vi "CloseMUXChannel.vi"(8 "error in (no error)":errorcluster, 10 "gRPCid":T2, 11 "ctet_mux in":T1) -> (0 "error out":errorcluster, 3 "ctet_mux out":T1)   [LabVIEW 2019, in "ctet_mux_User Library.lvlib"]
uses:
  ctet_mux_User Library.lvlib
  Servers/ctet_mux/gRPC lvSupport/Server API/typeDefs/grpcId.ctl
  Types/ctet_mux.ctl
  Servers/ctet_mux/ctet_mux Class/RPC Messages/measurementservice_MUXCloseChannelResponse/measurementservice_MUXCloseChannelResponse_Data.ctl
  Servers/ctet_mux/ctet_mux Class/RPC Messages/measurementservice_ErrorOut/measurementservice_ErrorOut_Data.ctl
  <instrlib>/niSwitch/niSwitch.llb/niSwitch Connect Channels (Single).vi
  Servers/ctet_mux/ctet_mux Class/ctet_mux.lvclass
  Servers/ctet_mux/gRPC lvSupport/gprc-lvsupport.lvlib
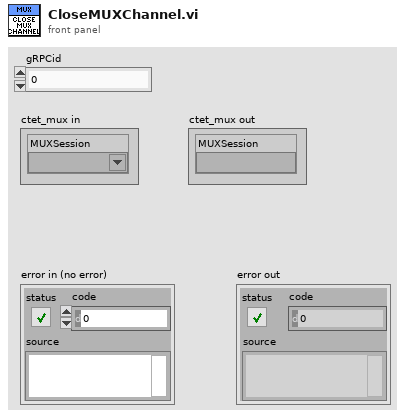
[diagram p1: front panel]
types:
  T1 = typedef "ctet_mux_User Library.lvlib/ctet_mux.ctl" = cluster{"MUXSession":refnum<k15>}
  T2 = typedef "ctet_mux.lvlib/gprc-lvsupport.lvlib/grpcId.ctl" = u64
  T3 = typedef "ctet_mux.lvlib/ctet_mux.lvclass/measurementservice_ErrorOut_Data.ctl" = cluster{"errCode":i64, "errMessage":string}
  T4 = typedef "ctet_mux.lvlib/ctet_mux.lvclass/measurementservice_MUXCloseChannelResponse_Data.ctl" = cluster{"error":T3}
  T5 = typedef "ctet_mux.lvlib/ctet_mux.lvclass/measurementservice_MUXCloseChannelRequest_Data.ctl" = cluster{"Channel1":string, "Channel2":string}
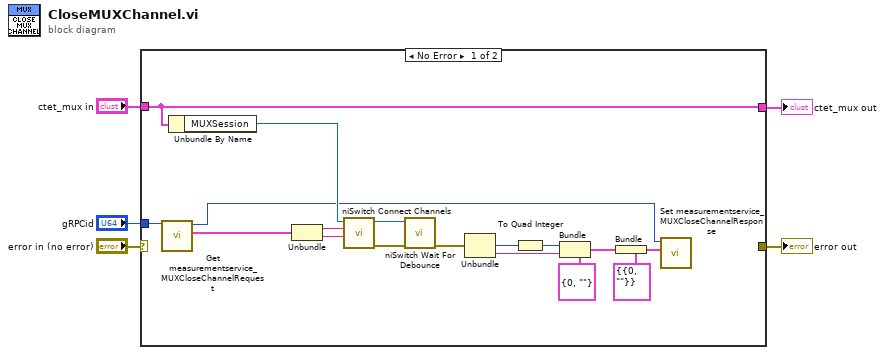
[diagram p0: block diagram]
diagram:
  n1 = case shown="No Error" "error in (no error)" {
    selector: "error in (no error)" -> [_ w24]
    tunnel: [_ w24] -> w5
    tunnel: "gRPCid" -> [w18 _]
    tunnel: "ctet_mux in" -> [w19 w23]
    tunnel: [w19 w23] -> w1
    frame No Error {
      n2 = call "Get measurementservice_MUXCloseChannelRequest.vi"("gRPCid"=w18) -> ("Message Data"=w17:T5, "gRPCid out"=w6:T2)  [unwired: 8 in, 1 out]
      n3 = Unbundle By Name(w19) -> ("MUXSession"=w9:refnum<k15>)
      n4 = Unbundle(w17) -> ("Channel1"=w8:string, "Channel2"=w7:string)
      n5 = call-poly <instrlib>:"niSwitch Connect Channels.vi"("channel 2"=w7, "channel 1"=w8, "instrument handle"=w9) -> ("error out"=w11:errorcluster, "instrument handle out"=w12:refnum<k15>)  [unwired: 7 in]
      n6 = call <instrlib>:"niSwitch Wait For Debounce.vi"("error in (no error)"=w11, "instrument handle"=w12) -> ("error out"=w10:errorcluster)  [unwired: 8 in, 1 out]
      n7 = Unbundle(w10) -> ("code"=w21:i32, "source"=w22:string)  [unwired: 1 out]
      n8 = To Quad Integer(1:w21) -> (0:w20:i64)
      n9 = Bundle(cluster=T3 {"errCode"=0, "errMessage"=""} ("error"), "errCode"=w20, "errMessage"=w22) -> (w13:T3)
      n10 = Bundle(cluster=T4 {"error"={"errCode"=0, "errMessage"=""}} ("Message Data"), "error"=w13) -> (w15:T4)
      n11 = call "Set measurementservice_MUXCloseChannelResponse.vi"("Message Data"=w15, "gRPCid"=w6) -> ()  [unwired: 9 in, 1 out]
    }
    frame Error {
    }
  }
  "error out" <- w5
  "ctet_mux out" <- w1
